vi "MAIN FPGA.vi"() -> ()   [LabVIEW 2019]
uses:
  TypeDef/FPGA AIs.ctl
  TypeDef/FPGA AI Loop Data.ctl
  TypeDef/FPGA DO Loop Data.ctl
  TypeDef/FPGA DI Loop Data.ctl
  <vilib>/rvi/Emulation/niFpgaGetClockAttributes.vi
  <vilib>/rvi/Emulation/niFpgaSctlEmulationGetInTimedLoop.vi
  <vilib>/rvi/Emulation/niFpgaEmulationReportErrorSimple.vi
  <vilib>/rvi/interface/RandomDataEmulation/niFpgaRandomDataHandleErrors.vi
  <vilib>/rvi/Emulation/niFpgaEmulationIsFPGAContextNoSignature.vi
  <vilib>/rvi/errors/niFpgaSetErrorForExecOnDevCompSimple.vi
  <vilib>/rvi/eio/common/nirviEmuReportErrorAndStop.vi
  <vilib>/rvi/DataTransferAndStorage/Container/Common/niFpgaContainerGetUniqueNameForEmu.vi
  <vilib>/rvi/FIFO/Fifo_Resource/nirvififoEmulationSetSize.vi
  <vilib>/rvi/FIFO/Fifo_Resource/nirviFifoEmulationQueueMgr.vi
  <instcachedir>/0/nirviFifoEmulationQueueMgr_E5CAEC123FF24DC58D834DCA3CDAA9B5.lvgen/nirviFifoEmulationQueueMgr_E5CAEC123FF24DC58D834DCA3CDAA9B5_002.vi
  <vilib>/rvi/FIFO/Fifo_Resource/nirvififoEmulationDetermineInputValidOut.vi
  <vilib>/rvi/FIFO/Fifo_Resource/nirvififoEmulationCreateLock.vi
  <vilib>/rvi/Emulation/niFpgaProcessEmulError.vi
  <vilib>/rvi/FIFO/Fifo_Resource/nirvififoEmulationObtainLock.vi
  <vilib>/rvi/FIFO/Fifo_Resource/nirvififoEmulationReleaseLock.vi
  <vilib>/rvi/occurrence/nirviWaitOnOccurrenceBase.vi
  <vilib>/rvi/errors/nirviReportUnexpectedCaseInternalError.vi
  <vilib>/rvi/errors/nirviReportUnexpectedCaseInternalError (U32).vi
  <vilib>/rvi/Emulation/niFpgaCriticalErrorInLSC.vi
  <vilib>/rvi/eio/common/nirviEmuTemplateMethod_errors.vi
  <vilib>/rvi/DataTransferAndStorage/Container/XNode/niFpgaContainer.xnode
  <vilib>/rvi/interface/RandomDataEmulation/nirviRandomDataFpgaReadWriteTemplate.vi
  <vilib>/rvi/FIFO/Fifo_Resource/nirvififoEmulationWrite.vi
  <vilib>/eio/EIONode/EIONode.xnode
panel:
  in  "Count(uSec)":u32=1000
  out "Mod5/AO1 out":fxp<+/-,20,5>
  in  "upper limit":fxp<+/-,21,6>=0.001007080078125
  in  "lower limit":fxp<+/-,21,6>=-1.0
  out "DO":u32
  out "Average 1ms":T1
  out "Raw":T1
  out "Error AO":errorcluster
  in  "Mod5/AO0":fxp<+/-,20,5>
  in  "Mod5/AO1":fxp<+/-,20,5>
  in  "Mod5/AO2":fxp<+/-,20,5>
  in  "Mod5/AO3":fxp<+/-,20,5>
  out "dt (ticks) AO Loop":u32
  out "DI":u32
  out "Error DI":errorcluster
  in  "Cycles to Filter DI":u16=100
  out "dt(tiks) DI loop":u32
  out "Error DO":errorcluster
  out "FIFO AI Timed Out?":bool
  out "Error AI mod 2":errorcluster
  out "Error AI mod 1":errorcluster
  out "dt(tiks) DO loop":u32
  out "dt(tiks) AI loop":u32
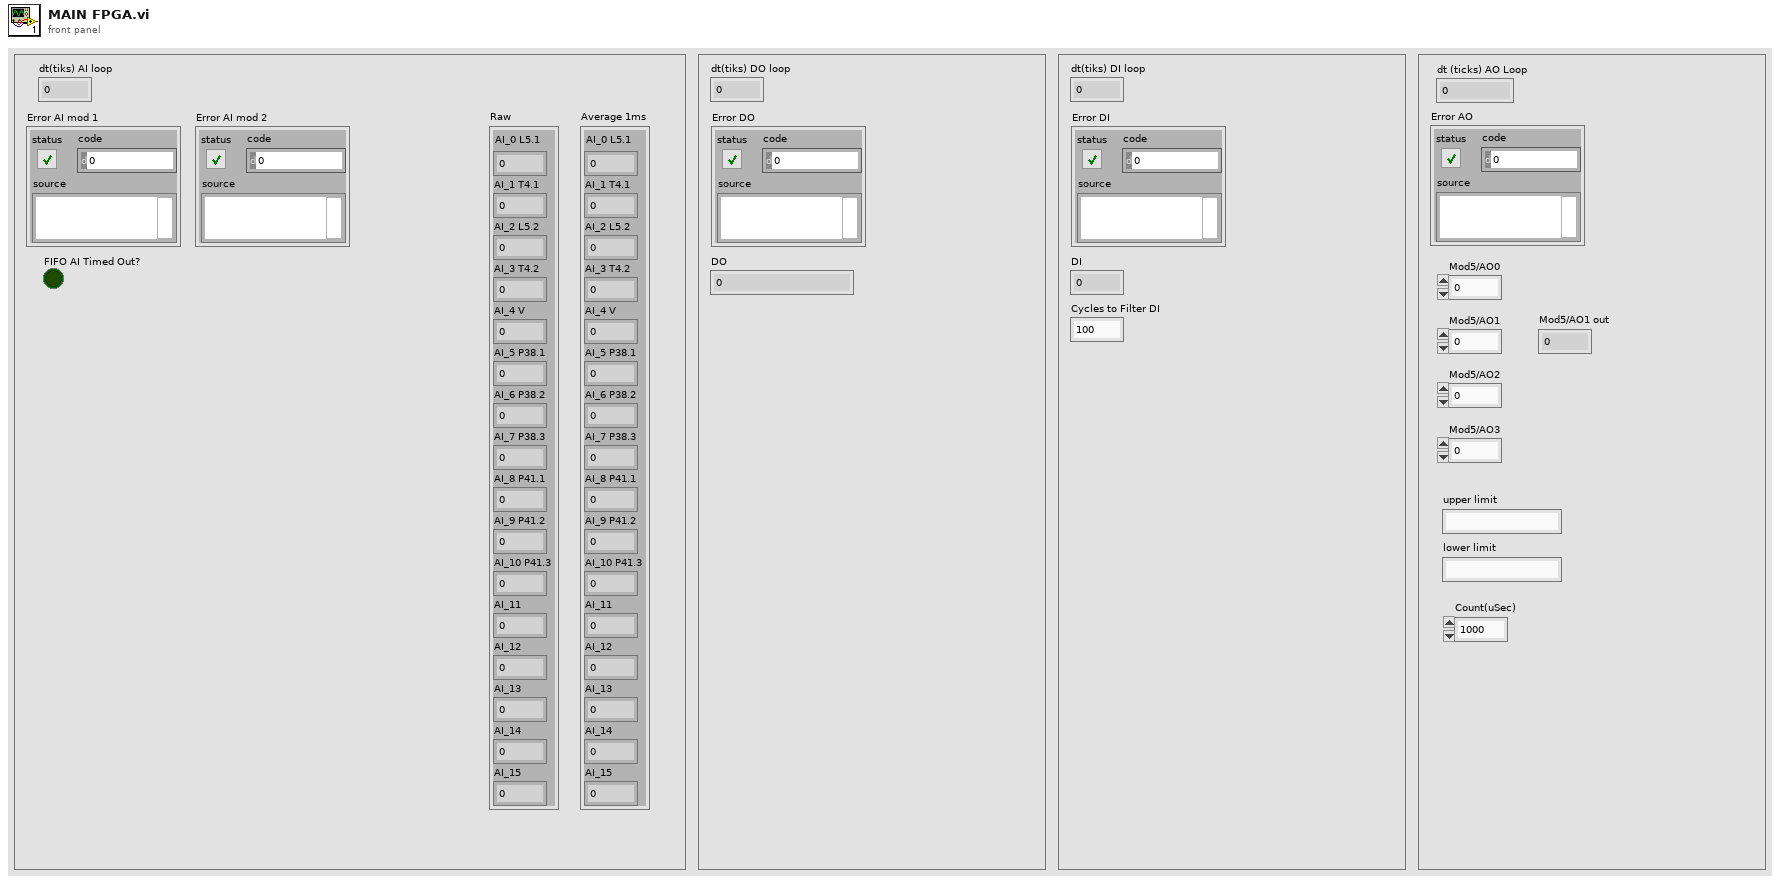
[diagram p1: front panel]
types:
  T1 = typedef "FPGA AIs.ctl" = cluster{"AI_0 L5.1":fxp<+/-,21,-4>, "AI_1 T4.1":fxp<+/-,21,-4>, "AI_2 L5.2":fxp<+/-,21,-4>, "AI_3 T4.2":fxp<+/-,21,-4>, "AI_4 V":fxp<+/-,21,-4>, "AI_5 P38.1":fxp<+/-,21,-4>, "AI_6 P38.2":fxp<+/-,21,-4>, "AI_7 P38.3":fxp<+/-,21,-4>, "AI_8 P41.1":fxp<+/-,21,-4>, "AI_9 P41.2":fxp<+/-,21,-4>, "AI_10 P41.3":fxp<+/-,21,-4>, "AI_11":fxp<+/-,21,-4>, "AI_12":fxp<+/-,21,-4>, "AI_13":fxp<+/-,21,-4>, "AI_14":fxp<+/-,21,-4>, "AI_15":fxp<+/-,21,-4>}
  T2 = typedef "FPGA DI Loop Data.ctl" = cluster{"DI":bool[], "Set Time uSec":u16[]}
  T3 = typedef "FPGA DO Loop Data.ctl" = cluster{"DO":bool[], "Is Pulse":bool[], "Set Time uSec":u32[], "Wait Time uSec":u32[]}
  T4 = typedef "FPGA AI Loop Data.ctl" = cluster{"Raw":T1, "Average 1ms":T1, "mean valid":bool}
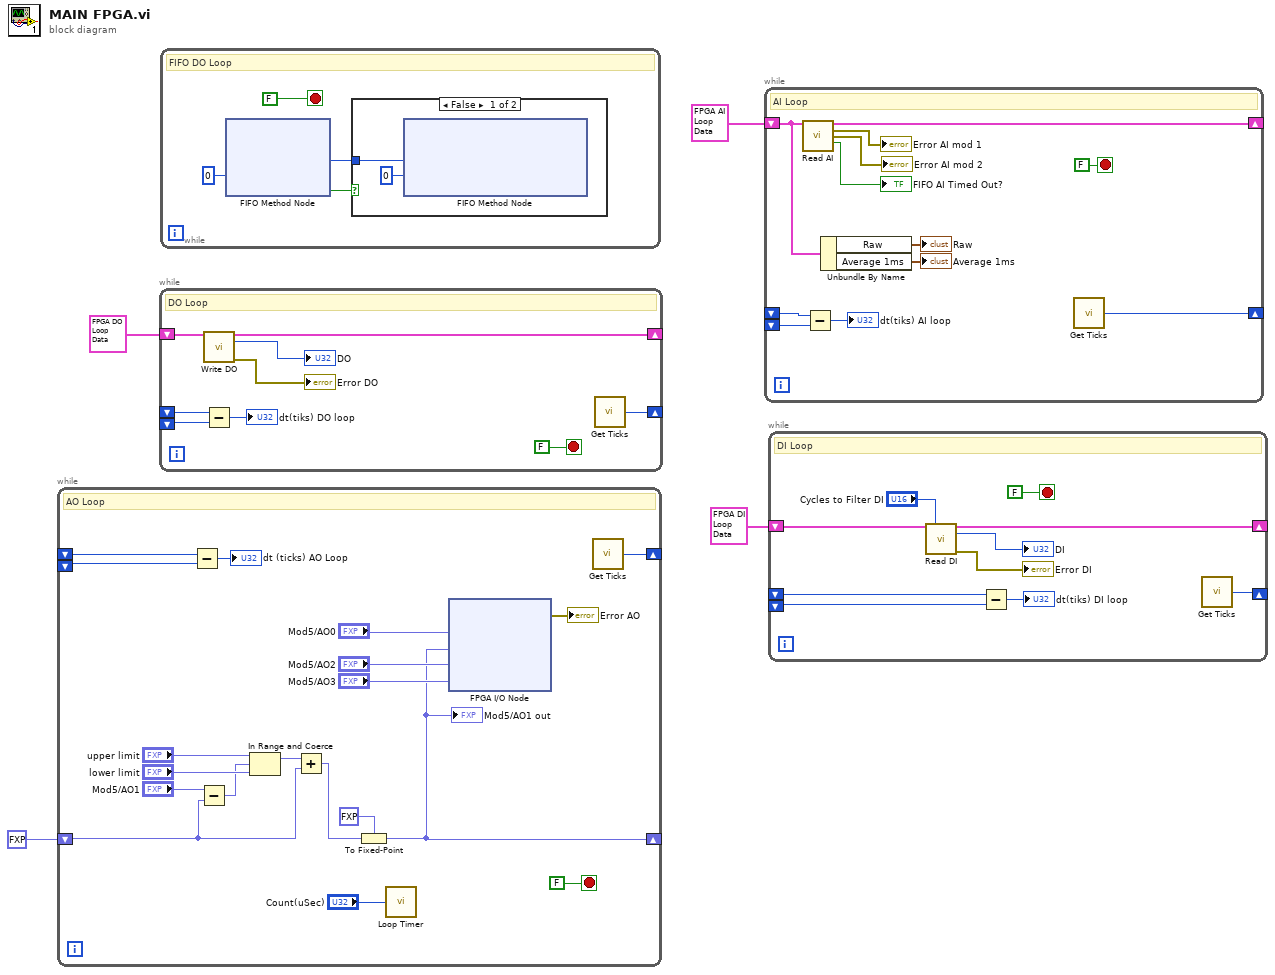
[diagram p0: block diagram]
diagram:
  n1 = while {
    shift-right: [w15] -> _
    shift-left: _ -> [w17]
    shift-left: _ -> [w16]
    shift-right: [w6] -> _
    shift-left: fxp<+/-,20,5> 0.0 ("Mod5/AO1") -> [w9]
    stop <- FALSE stop-if-true
    # "AO Loop"
    n2 = Subtract(x=w17, y=w16) -> (x-y=→"dt (ticks) AO Loop":u32)
    n3 = Subtract(x="Mod5/AO1", y=w9) -> (x-y=w10:fxp<+/-,21,6>)
    n4 = In Range and Coerce(upper limit="upper limit", x=w10, lower limit="lower limit") -> (coerced(x)=w12:fxp<+/-,21,6>)  [unwired: 1 out]
    n5 = Add(x=w12, y=w9) -> (x+y=w7:fxp<+/-,22,7>)
    n6 = To Fixed-Point(fixed-point type=fxp<+/-,20,5> 0.0 ("Mod5/AO1"), number=w7) -> (fixed-point=w6:fxp<+/-,20,5>)
    "Mod5/AO1 out" <- w6
    n7 = call "Loop Timer"("Count(uSec)"="Count(uSec)") -> ()  [unwired: 1 out]
    n8 = xnode "FPGA I/O Node"("Mod5/AO0"="Mod5/AO0", "Mod5/AO1"=w6, "Mod5/AO2"="Mod5/AO2", "Mod5/AO3"="Mod5/AO3") -> ("error out"=→"Error AO":errorcluster)  [unwired: 5 in, 4 out]
    n9 = call "Get Ticks.vi"() -> ("Tick Count(Ticks)"=w15:u32)
  }
  n10 = while {
    shift-right: [w27] -> _
    shift-left: T3 {"DO"=[FALSE, FALSE, FALSE, FALSE, FALSE, FALSE, FALSE, FALSE, FALSE, FALSE, FALSE, FALSE, FALSE, FALSE, FALSE, FALSE, FALSE, FALSE, FALSE, FALSE, FALSE, FALSE, FALSE, FALSE, FALSE, FALSE, FALSE, FALSE, FALSE, FALSE, FALSE, FALSE], "Is Pulse"=[FALSE, FALSE, FALSE, FALSE, FALSE, FALSE, FALSE, FALSE, FALSE, FALSE, FALSE, FALSE, FALSE, FALSE, FALSE, FALSE, FALSE, FALSE, FALSE, FALSE, FALSE, FALSE, FALSE, FALSE, FALSE, FALSE, FALSE, FALSE, FALSE, FALSE, FALSE, FALSE], "Set Time uSec"=[0, 0, 0, 0, 0, 0, 0, 0, 0, 0, 0, 0, 0, 0, 0, 0, 0, 0, 0, 0, 0, 0, 0, 0, 0, 0, 0, 0, 0, 0, 0, 0], "Wait Time uSec"=[0, 0, 0, 0, 0, 0, 0, 0, 0, 0, 0, 0, 0, 0, 0, 0, 0, 0, 0, 0, 0, 0, 0, 0, 0, 0, 0, 0, 0, 0, 0, 0]} ("FPGA DO Loop Data") -> [w28]
    shift-right: [w25] -> _
    shift-left: _ -> [w30]
    shift-left: _ -> [w29]
    stop <- FALSE stop-if-true
    # "DO Loop"
    n11 = call "Write DO.vi"("FPGA DO Loop Data in"=w28) -> ("FPGA DO Loop Data out"=w27:T3, "DO"=→"DO":u32, "error out"=→"Error DO":errorcluster)  [unwired: 12 in]
    n12 = Subtract(x=w30, y=w29) -> (x-y=→"dt(tiks) DO loop":u32)
    n13 = call "Get Ticks.vi"() -> ("Tick Count(Ticks)"=w25:u32)
  }
  n14 = while {
    stop <- FALSE stop-if-true
    # "FIFO DO Loop"
    n15 = xnode ("FIFO Method Node")("Timeout"=0) -> ("Element"=w33:u64, "Timed Out?"=w34:bool)  [unwired: 1 in, 1 out]
    n16 = case shown="False" w34 {
      tunnel: w33 -> [w38 _]
      frame False {
        n17 = xnode ("FIFO Method Node")("Element"=w38, "Timeout"=0) -> ()  [unwired: 1 in, 2 out]
      }
      frame True {
      }
    }
  }
  n18 = while {
    shift-right: [w39] -> _
    shift-left: T4 {"Raw"={"AI_0 L5.1"=0.0, "AI_1 T4.1"=0.0, "AI_2 L5.2"=0.0, "AI_3 T4.2"=0.0, "AI_4 V"=0.0, "AI_5 P38.1"=0.0, "AI_6 P38.2"=0.0, "AI_7 P38.3"=0.0, "AI_8 P41.1"=0.0, "AI_9 P41.2"=0.0, "AI_10 P41.3"=0.0, "AI_11"=0.0, "AI_12"=0.0, "AI_13"=0.0, "AI_14"=0.0, "AI_15"=0.0}, "Average 1ms"={"AI_0 L5.1"=0.0, "AI_1 T4.1"=0.0, "AI_2 L5.2"=0.0, "AI_3 T4.2"=0.0, "AI_4 V"=0.0, "AI_5 P38.1"=0.0, "AI_6 P38.2"=0.0, "AI_7 P38.3"=0.0, "AI_8 P41.1"=0.0, "AI_9 P41.2"=0.0, "AI_10 P41.3"=0.0, "AI_11"=0.0, "AI_12"=0.0, "AI_13"=0.0, "AI_14"=0.0, "AI_15"=0.0}, "mean valid"=FALSE} ("FPGA AI Loop Data in") -> [w43]
    shift-right: [w40] -> _
    shift-left: _ -> [w49]
    shift-left: _ -> [w48]
    stop <- FALSE stop-if-true
    # "AI Loop"
    n19 = call "Read AI.vi"("FPGA AI Loop Data in"=w43) -> ("FPGA AI Loop Data out"=w39:T4, "Error AI mod 1"=→"Error AI mod 1":errorcluster, "Error AI mod 2"=→"Error AI mod 2":errorcluster, "FIFO AI Timed Out?"=→"FIFO AI Timed Out?":bool)  [unwired: 11 in]
    n20 = Subtract(x=w49, y=w48) -> (x-y=→"dt(tiks) AI loop":u32)
    n21 = Unbundle By Name(w43) -> ("Raw"=→"Raw":T1, "Average 1ms"=→"Average 1ms":T1)
    n22 = call "Get Ticks.vi"() -> ("Tick Count(Ticks)"=w40:u32)
  }
  n23 = while {
    shift-right: [w55] -> _
    shift-left: T2 {"DI"=[FALSE, FALSE, FALSE, FALSE, FALSE, FALSE, FALSE, FALSE, FALSE, FALSE, FALSE, FALSE, FALSE, FALSE, FALSE, FALSE, FALSE, FALSE, FALSE, FALSE, FALSE, FALSE, FALSE, FALSE, FALSE, FALSE, FALSE, FALSE, FALSE, FALSE, FALSE, FALSE], "Set Time uSec"=[0, 0, 0, 0, 0, 0, 0, 0, 0, 0, 0, 0, 0, 0, 0, 0, 0, 0, 0, 0, 0, 0, 0, 0, 0, 0, 0, 0, 0, 0, 0, 0]} ("FPGA DI Loop Data") -> [w59]
    shift-right: [w51] -> _
    shift-left: _ -> [w57]
    shift-left: _ -> [w56]
    stop <- FALSE stop-if-true
    # "DI Loop"
    n24 = call "Read DI.vi"("FPGA DI Loop Data in"=w59, "Cycles to Filter"="Cycles to Filter DI") -> ("FPGA DI Loop Data out"=w55:T2, "DI"=→"DI":u32, "error out"=→"Error DI":errorcluster)  [unwired: 11 in]
    n25 = Subtract(x=w57, y=w56) -> (x-y=→"dt(tiks) DI loop":u32)
    n26 = call "Get Ticks.vi"() -> ("Tick Count(Ticks)"=w51:u32)
  }
